vi "format display.vi"(6 "Channel":dbl(slide)=1.0 min=0.0 max=7.0 step=1.0 scale=0.0..7.0, 9 "Display":enum16{"X and Y", "R and Theta"}(ring), 10 "Results (X,Y,R,Theta)":dbl[][](array[numeric]), 11 "t0":timestamp) -> (0 "X/R":dbl, 1 "Array 2":cluster{dbl[], dbl[]}[](array[cluster]), 2 "Y/Theta Array":waveform(dbl)[](array[waveform]), 3 "X/R Array":waveform(dbl)[](array[waveform]), 4 "Y/R":dbl)   [LabVIEW 2016]
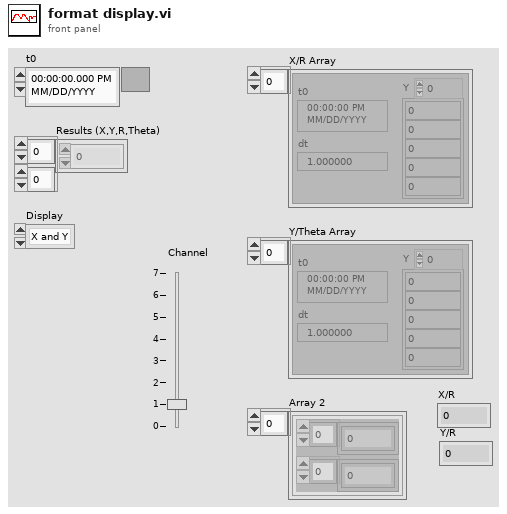
[diagram p1: front panel]
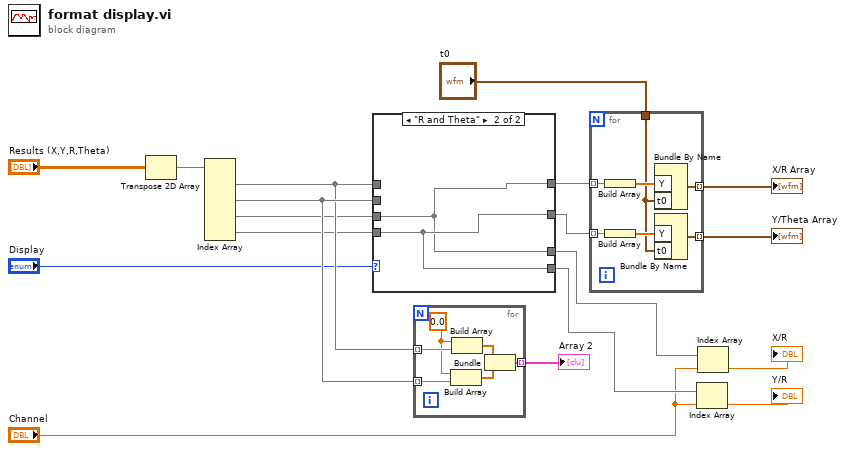
[diagram p0: block diagram]
diagram:
  n1 = Transpose 2D Array(2D array="Results (X,Y,R,Theta)") -> (transposed array=w8:dbl[][])
  n2 = Index Array(array=w8) -> (element #1=w15:dbl[], element #2=w16:dbl[], element #3=w11:dbl[], element #4=w12:dbl[])  [unwired: 8 in]
  n3 = case shown="\"R and Theta\"" "Display" {
    tunnel: w15 -> [w19 _]
    tunnel: [w19 w21] -> w7
    tunnel: w16 -> [w20 _]
    tunnel: [w20 w22] -> w6
    tunnel: w11 -> [_ w21]
    tunnel: w12 -> [_ w22]
    tunnel: [w20 w22] -> w2
    tunnel: [w19 w21] -> w3
    frame "X and Y", Default {
    }
    frame "R and Theta" {
    }
  }
  n4 = for {
    tunnel: w15 -> [w28] mode=indexing
    tunnel: w16 -> [w27] mode=indexing
    tunnel: [w23] -> w17 mode=indexing
    w26 = 0.0
    n5 = Build Array(w26, w27) -> (w24:dbl[])
    n6 = Build Array(w26, w28) -> (w25:dbl[])
    n7 = Bundle(w25, w24) -> (w23:cluster{dbl[], dbl[]})  [unwired: 1 in]
  }
  "Array 2" <- w17
  n8 = for {
    tunnel: w7 -> [w35] mode=indexing
    tunnel: w6 -> [w34] mode=indexing
    tunnel: [w33] -> w14 mode=indexing
    tunnel: [w32] -> w18 mode=indexing
    tunnel: "t0" -> [w29]
    n9 = Build Array(w35) -> (w31:dbl[])
    n10 = Build Array(w34) -> (w30:dbl[])
    n11 = Bundle By Name("Y"=w31, "t0"=w29) -> (w33:waveform(dbl))  [unwired: 1 in]
    n12 = Bundle By Name("Y"=w30, "t0"=w29) -> (w32:waveform(dbl))  [unwired: 1 in]
  }
  "Y/Theta Array" <- w18
  "X/R Array" <- w14
  n13 = Index Array(array=w2, index="Channel") -> (element=→"Y/R":dbl)
  n14 = Index Array(array=w3, index="Channel") -> (element=→"X/R":dbl)
